vi "SPADQ_AcquisitionStatus.vi"(6 "WaitTime (ms)":dbl, 8 "error in (no error)":errorcluster, 9 "adq_num":i32, 10 "adq_cu_ptr in":refnum<k24>, 11 "ADQAPI Ref":refnum<k24>) -> (0 "error out":errorcluster, 1 "Error Text":string, 2 "return":i32, 3 "ADQAPI Ref (out)":refnum<k24>)   [LabVIEW 2022 SP3]
doc: "_____AlazarTech, Scope_____\n\nSet the Trigger delay"
uses:
  C:/Windows/System32/ADQAPI_dotNet_helper.dll
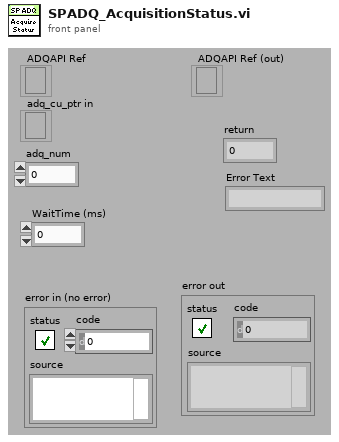
[diagram p1: front panel]
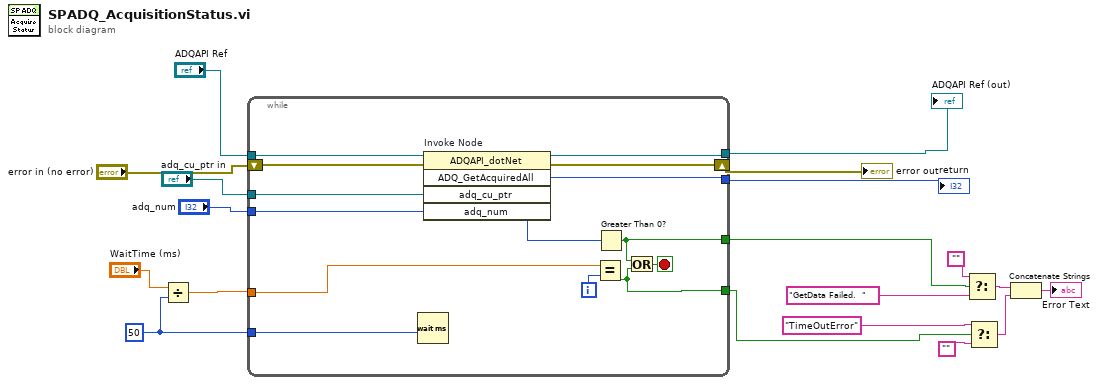
[diagram p0: block diagram]
diagram:
  w1 = u32 50 ("milliseconds to wait")
  n1 = Divide(x="WaitTime (ms)", y=w1) -> (x/y=w12:dbl)
  n2 = while {
    tunnel: [w30] -> w4
    tunnel: [w29] -> w5
    tunnel: "ADQAPI Ref" -> [w28]
    tunnel: "adq_cu_ptr in" -> [w26]
    tunnel: "adq_num" -> [w25]
    tunnel: [w24] -> w15
    tunnel: [w22] -> w13
    shift-right: [w23] -> w14
    shift-left: "error in (no error)" -> [w27]
    tunnel: w12 -> [w21]
    tunnel: w1 -> [w20]
    i -> [w32]
    stop <- w31 stop-if-true
    n3 = Wait (ms)(milliseconds to wait=w20) -> ()  [unwired: 1 out]
    n4 = invoke on="Invoke Node" class="ADQAPI_dotNet" method="ADQ_GetAcquiredAll"(reference=w28, error in=w27, "adq_cu_ptr"=w26, "adq_num"=w25) -> (reference out=w24:refnum<k24>, error out=w23:errorcluster, "ADQ_GetAcquiredAll"=w22:u32)  [unwired: 1 in, 2 out]
    n5 = Equal?(x=w21, y=w32) -> (x = y?=w30:bool)
    n6 = Greater Than 0?(x=w22) -> (x > 0?=w29:bool)
    n7 = Or(x=w29, y=w30) -> (x .or. y?=w31:bool)
  }
  "error out" <- w14
  "ADQAPI Ref (out)" <- w15
  "return" <- w13
  n8 = Select(t="", s=w5, f="GetData Failed.  ") -> (s? t:f=w7:string)
  n9 = Select(t="TimeOutError", s=w4, f="") -> (s? t:f=w6:string)
  n10 = Concatenate Strings(w7, w6) -> (→"Error Text":string)
